vi "数组相加.vi"() -> ()   [LabVIEW 2020]
doc: "本VI是为《我和LabVIEW》一书编写的示例。\n关于本书的介绍请参考网页：\nhttp://ruanqizhen.spaces.live.com/blog/cns!5852D4F797C53FB6!4310.entry"
panel:
  in  "数组 b":i32[](array[numeric])
  out "结果 2":i32[](array[numeric])
  in  "数组 a":i32[](array[numeric])
  out "结果":i32[](array[numeric])
  in  "数值":i32
  in  "数组":i32[](array[numeric])
  # "+"
  # "="
  # "+"
  # "="
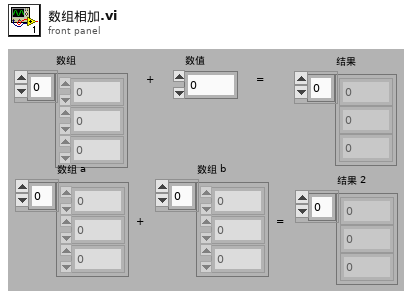
[diagram p1: front panel]
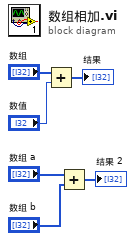
[diagram p0: block diagram]
diagram:
  n1 = Add(x="数组", y="数值") -> (x+y=→"结果":i32[])
  n2 = Add(x="数组 a", y="数组 b") -> (x+y=→"结果 2":i32[])
